vi "Visualize Image.vi"(11 "Puzzle 20-1":T1) -> (3 "Image":i16[][](graph))   [LabVIEW 2020]
uses:
  Puzzle 20-1.ctl
  Vec2.ctl
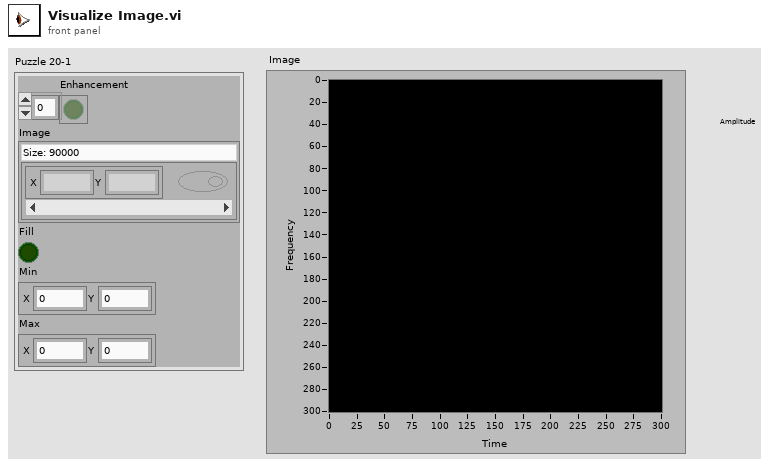
[diagram p1: front panel]
types:
  T1 = typedef "Puzzle 20-1.ctl" = cluster{"Enhancement":bool[], "Image":map{T2, bool}, "Fill":bool, "Min":T2, "Max":T2}
  T2 = typedef "Vec2.ctl" = cluster{"X":i32, "Y":i32}
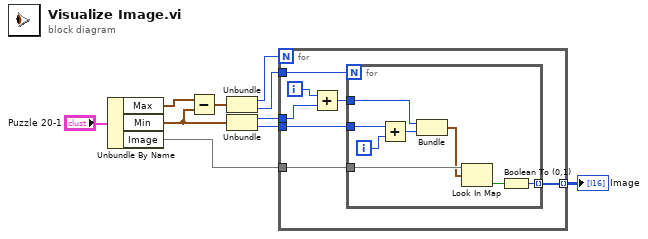
[diagram p0: block diagram]
diagram:
  n1 = Unbundle By Name("Puzzle 20-1") -> ("Max"=w9:T2, "Min"=w7:T2, "Image"=w6:map{T2, bool})
  n2 = Subtract(x=w9, y=w7) -> (x-y=w8:T2)
  n3 = Unbundle(w8) -> ("X"=w5:i32, "Y"=w4:i32)
  n4 = Unbundle(w7) -> ("X"=w3:i32, "Y"=w2:i32)
  n5 = for {
    N: w5 -> [_]
    tunnel: w6 -> [w12]
    tunnel: w4 -> [w17]
    tunnel: w3 -> [w15]
    tunnel: w2 -> [w16]
    tunnel: [w11] -> w1 mode=indexing
    i -> [w14]
    n6 = Add(x=w14, y=w15) -> (x+y=w13:i32)
    n7 = for {
      N: w17 -> [_]
      tunnel: w16 -> [w25]
      tunnel: w13 -> [w23]
      tunnel: w12 -> [w21]
      tunnel: [w18] -> w11 mode=indexing
      i -> [w24]
      n8 = Add(x=w25, y=w24) -> (x+y=w22:i32)
      n9 = Bundle(w23, w22) -> (w20:cluster{i32, i32})  [unwired: 1 in]
      n10 = Look In Map(map=w21, key=w20) -> (value=w19:bool)  [unwired: 1 in, 1 out]
      n11 = Boolean To (0,1)(Boolean=w19) -> (0, 1=w18:i16)
    }
  }
  "Image" <- w1
